vi "Decode float.vi"(10 "Wire Type":T1=enum."I32", 11 "Data":u8[](array[numeric]) format="%.0x") -> (2 "error out":errorcluster, 3 "float":sgl)   [LabVIEW 2020, in "LV-Proto.lvlib"]
uses:
  LV-Proto.lvlib
  Wire Type.ctl
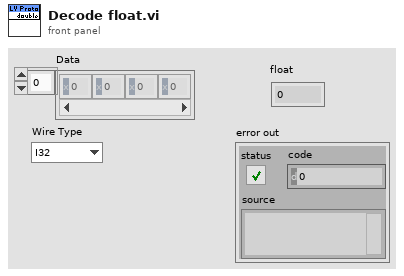
[diagram p1: front panel]
types:
  T1 = typedef "LV-Proto.lvlib/Wire Type.ctl" = enum8{"VARINT", "I64", "LEN", "SGROUP (Deprecated)", "EGROUP (Deprecated)", "I32"}
  T2 = enum16{"big-endian, network order", "native, host order", "little-endian"}
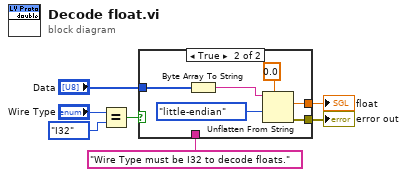
[diagram p0: block diagram]
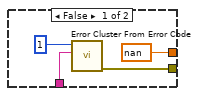
[diagram p2: hidden frame]
diagram:
  n1 = Equal?(x="Wire Type", y=Wire_Type."I32") -> (x = y?=w3:bool)
  n2 = case shown="True" w3 {
    tunnel: "Data" -> [_ w17]
    tunnel: [sgl nan w14] -> w6
    tunnel: [w10 w13] -> w2
    tunnel: "Wire Type must be I32 to decode floats." -> [w8 _]
    frame False {
      n3 = call <vilib>:"Error Cluster From Error Code.vi"("error message (\"\")"=w8, "error code (0)"=1) -> ("error out"=w10:errorcluster)  [unwired: 7 in]
    }
    frame True {
      n4 = Byte Array To String(unsigned byte array=w17) -> (string=w12:string)
      n5 = Unflatten From String(type=sgl 0.0, binary string=w12, byte order (0:big-endian, network order)=T2."little-endian") -> (value=w14:sgl, error out=w13:errorcluster)  [unwired: 2 in, 1 out]
    }
  }
  "float" <- w6
  "error out" <- w2
